vi "Controls - Memory.vi"(7 "Msg Chain":string, 8 "error in (no error)":errorcluster {"code" format="Error %.0f"}, 10 "Controls Docs":refnum<class "GUI Documentation.lvclass">[](array[class]), 11 "VIDoc Printer - Confluence In":refnum<class "VIDoc Printer - Confluence.lvclass">) -> (0 "error out":errorcluster {"code" format="Error %.0f"}, 3 "VIDoc Printer - Confluence Out":refnum<class "VIDoc Printer - Confluence.lvclass">)   [LabVIEW 2023, in "VIDoc Printer - Confluence.lvlib" / "VIDoc Printer - Confluence.lvclass"]
uses:
  VIDoc Printer - Confluence.lvclass
  Parsing/GUI Documentation/GUI Documentation.lvclass
  Confluence Formatting/Types/Format Combo Box.ctl
  Parsing/GUI Documentation/Get Total Data Size.vi
  VIDoc Printer - Confluence.lvclass/VIDoc Printer - Confluence.ctl
  Confluence Formatting/Confluence Formatting.lvlib
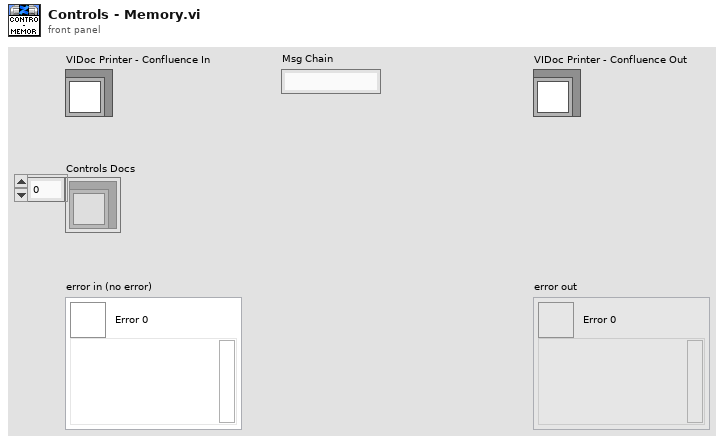
[diagram p1: front panel]
types:
  T1 = typedef "Confluence Formatting.lvlib/Format Combo Box.ctl" = string
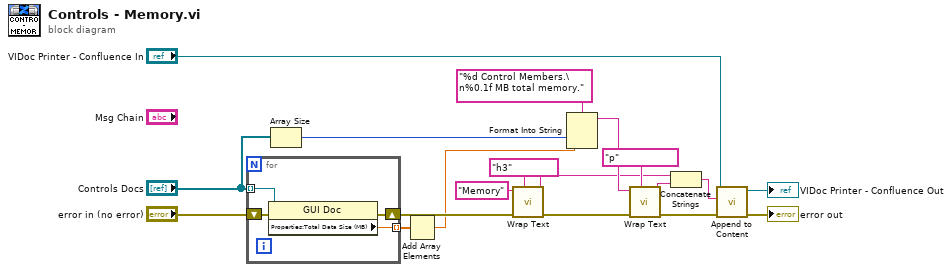
[diagram p0: block diagram]
diagram:
  n1 = for {
    tunnel: "Controls Docs" -> [w22] mode=indexing
    tunnel: [w21] -> w15 mode=indexing
    shift-right: [w20] -> w14
    shift-left: "error in (no error)" -> [w23]
    n2 = property class="GUI Doc"(reference=w22, error in=w23) -> (error out=w20:errorcluster, "Properties:Total Data Size (MB)"=w21:dbl)  [unwired: 1 out]
  }
  n3 = Array Size(array="Controls Docs") -> (size(s)=w7:i32)
  n4 = Add Array Elements(numeric array=w15) -> (sum=w6:dbl)
  n5 = call "Wrap Text.vi"("Formatting"=T1 "h3", "Error in"=w14, "String"="Memory") -> ("Error out"=w17:errorcluster, "Wrapped String"=w10:string)  [unwired: 7 in]
  n6 = Format Into String(format string="%d Control Members.\n%0.1f MB total memory.", w7, w6) -> (resulting string=w12:string)  [unwired: 2 in, 1 out]
  n7 = call "Wrap Text.vi"("Formatting"=T1 "p", "Error in"=w17, "String"=w12) -> ("Error out"=w16:errorcluster, "Wrapped String"=w9:string)  [unwired: 7 in]
  n8 = Concatenate Strings(w10, w9) -> (w8:string)
  n9 = call "Append to Content.vi"("error in (no error)"=w16, "Content"=w8, "VIDoc Printer - Confluence In"="VIDoc Printer - Confluence In") -> ("error out"=→"error out":errorcluster, "VIDoc Printer - Confluence Out"=→"VIDoc Printer - Confluence Out":refnum<class "VIDoc Printer - Confluence.lvclass">)  [unwired: 7 in]
